vi "03_1.vi"(10 "Increment":cluster{"Row":i32, "Column":i32}={"Row"=1, "Column"=3}, 11 "String":string) -> (3 "size(s)":i32)   [LabVIEW 2018]
uses:
  <userlib>/_OpenG.lib/array/array.llb/Search 1D Array (String)__ogtk.vi
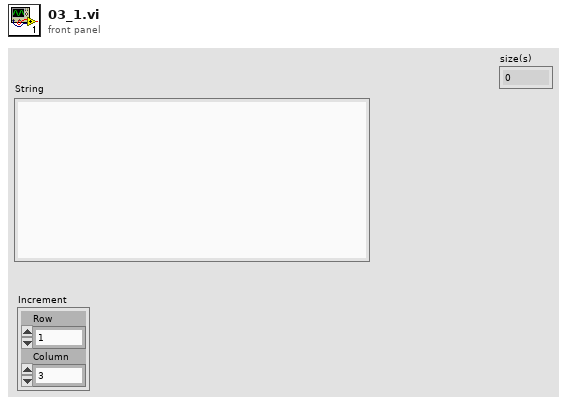
[diagram p1: front panel]
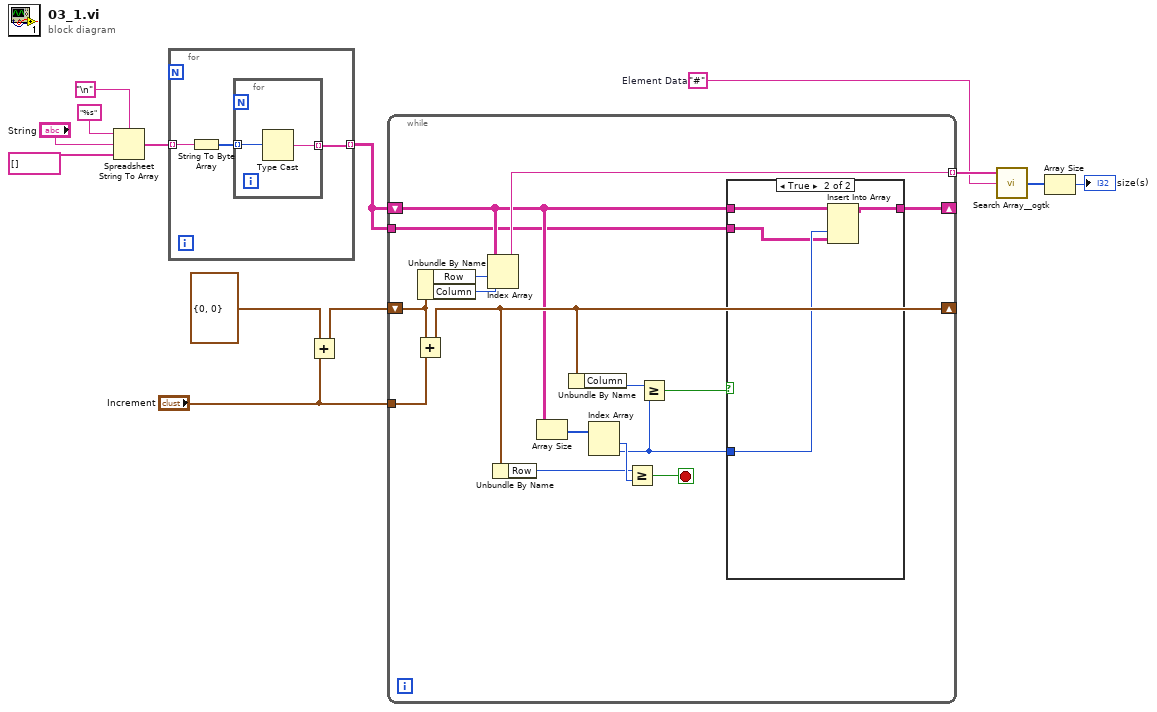
[diagram p0: block diagram]
diagram:
  w1 = "#"  # Element Data
  n1 = Spreadsheet String To Array(delimiter (Tab)="\n", format string="%s", spreadsheet string="String", array type (2D Dbl)=string[] []) -> (array=w3:string[])
  n2 = for {
    tunnel: w3 -> [w16] mode=indexing
    tunnel: [w14] -> w2 mode=indexing
    n3 = String To Byte Array(string=w16) -> (unsigned byte array=w15:u8[])
    n4 = for {
      tunnel: w15 -> [w18] mode=indexing
      tunnel: [w17] -> w14 mode=indexing
      n5 = Type Cast(x=w18) -> (*(type *) &x=w17:string)  [unwired: 1 in]
    }
  }
  n6 = Add(x=cluster{"Row":i32, "Column":i32} {"Row"=0, "Column"=0}, y="Increment") -> (x+y=w7:cluster{"Row":i32, "Column":i32})
  n7 = while {
    shift-right: [w21] -> _
    shift-left: w2 -> [w22]
    tunnel: w2 -> [w19]
    shift-right: [w25] -> _
    shift-left: w7 -> [w29]
    tunnel: "Increment" -> [w30]
    tunnel: [w26] -> w6 mode=indexing
    stop <- w27 stop-if-true
    n8 = Add(x=w29, y=w30) -> (x+y=w25:cluster{"Row":i32, "Column":i32})
    n9 = Unbundle By Name(w29) -> ("Row"=w31:i32, "Column"=w34:i32)
    n10 = Index Array(array=w22, index (row)=w31, index (col)=w34) -> (element=w26:string)
    n11 = Unbundle By Name(w25) -> ("Row"=w28:i32)
    n12 = Array Size(array=w22) -> (size(s)=w33:i32[])
    n13 = Unbundle By Name(w25) -> ("Column"=w24:i32)
    n14 = Index Array(array=w33) -> (element #1=w32:i32, element #2=w20:i32)  [unwired: 2 in]
    n15 = Greater Or Equal?(x=w28, y=w32) -> (x >= y?=w27:bool)
    n16 = Greater Or Equal?(x=w24, y=w20) -> (x >= y?=w23:bool)
    n17 = case shown="True" w23 {
      tunnel: w22 -> [w35 w39]
      tunnel: [w35 w36] -> w21
      tunnel: w20 -> [_ w38]
      tunnel: w19 -> [_ w37]
      frame False {
      }
      frame True {
        n18 = Insert Into Array(array=w39, index (col)=w38, new element=w37) -> (w36:string[][])  [unwired: 1 in]
      }
    }
  }
  n19 = call-poly <userlib>:"Search Array__ogtk.vi"("Array"=w6, "Element Data"=w1) -> ("Indices of Elements"=w5:i32[])  [unwired: 7 in]
  n20 = Array Size(array=w5) -> (size(s)=→"size(s)":i32)
